vi "JerarquiaOperaciones.vi"() -> ()   [LabVIEW 2015]
panel:
  in  "y":dbl=54.0
  in  "x":dbl=12.0
  out "x^2":dbl=144.0
  out "sqrt(x)":dbl=3.4641016151377544
  out "x/y":dbl=0.2222222222222222
  out "x*y":dbl=648.0
  out "x-y":dbl=-42.0
  out "x+y":dbl=66.0
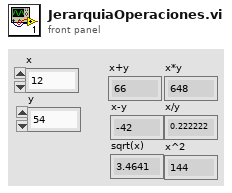
[diagram p1: front panel]
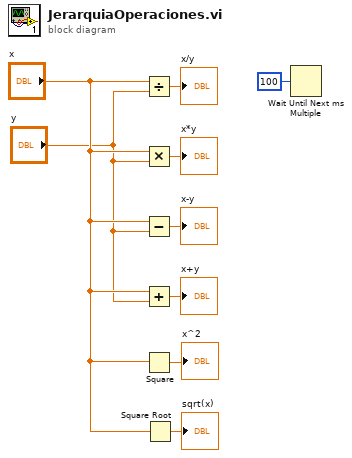
[diagram p0: block diagram]
diagram:
  n1 = Divide(x="x", y="y") -> (x/y=→"x/y":dbl)
  n2 = Multiply(x="x", y="y") -> (x*y=→"x*y":dbl)
  n3 = Subtract(x="x", y="y") -> (x-y=→"x-y":dbl)
  n4 = Add(x="x", y="y") -> (x+y=→"x+y":dbl)
  n5 = Square(x="x") -> (x^2=→"x^2":dbl)
  n6 = Square Root(x="x") -> (sqrt(x)=→"sqrt(x)":dbl)
  n7 = Wait Until Next ms Multiple(millisecond multiple=u32 100) -> ()  [unwired: 1 out]
